vi "edit_configurations.vi"() -> ()   [LabVIEW 2010]
uses:
  main/labview_source/type_definitions/classes/GenericPlugin/GenericPlugin.lvclass
  main/labview_source/type_definitions/clusters/plugin_specification.ctl
panel:
  in  "new":bool
  in  "Name":string
  in  "configure":bool
  in  "done":bool
  in  "Configuration":string(combo)
  in  "Path":path
  # "Edit existing configuration"
  # "create new configuration"
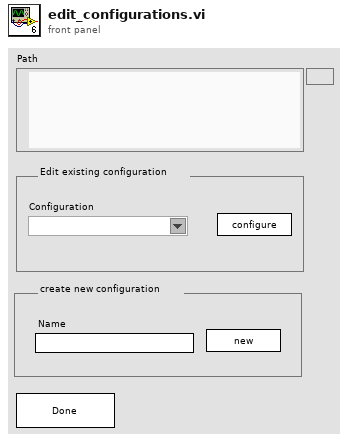
[diagram p1: front panel]
types:
  T1 = typedef "plugin_specification.ctl" = cluster{"class path":path, "configuration":string, "label":string}
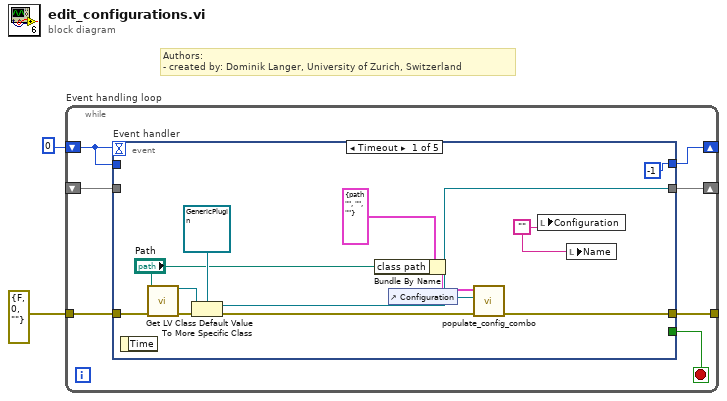
[diagram p0: block diagram]
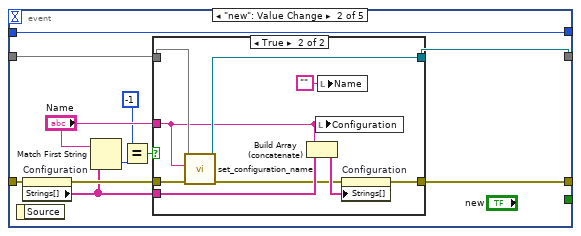
[diagram p2: hidden frame]
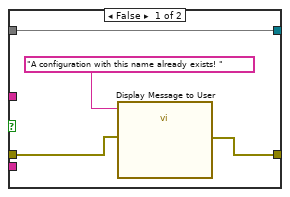
[diagram p3: hidden frame]
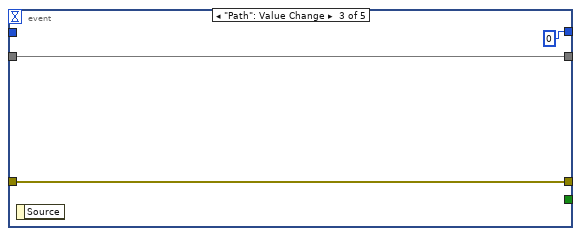
[diagram p4: hidden frame]
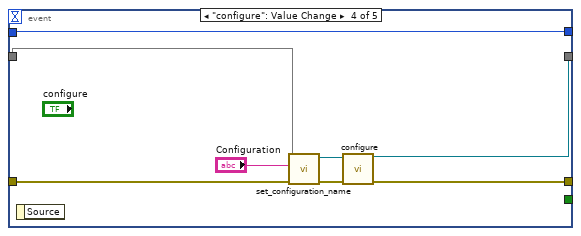
[diagram p5: hidden frame]
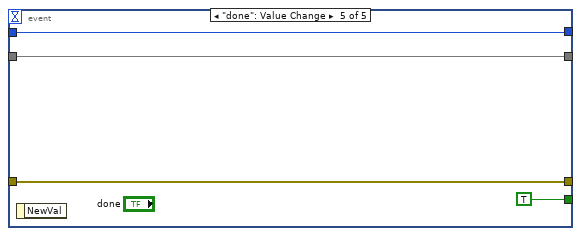
[diagram p6: hidden frame]
diagram:
  # "Authors: \n- created by: Dominik Langer, University of Zurich, Switzerland"
  n1 = while "Event handling loop" {
    shift-right: [w8] -> _
    shift-left: 0 -> [w9]
    shift-right: [w5] -> _
    shift-left: _ -> [w4]
    tunnel: errorcluster {"status"=FALSE, "code"=0, "source"=""} ("error in (no error)") -> [w6]
    tunnel: [w3] -> _
    stop <- w7 stop-if-true
    n2 = event "Event handler" shown="[0] Timeout" {
      selector: _ -> [_ _ _ _ _]
      dyn-events: _ -> [_ _ _ _ _]
      timeout: w9 -> [_ _ _ _ _]
      tunnel: w9 -> [_ w30 _ w52 w61]
      tunnel: [-1 w30 0 w52 w61] -> w8
      tunnel: [_ _ _ _ TRUE] -> w7
      tunnel: w6 -> [w21 w29 w47 w57 w58]
      tunnel: [w17 w32 w48 w53 w59] -> w5
      tunnel: w4 -> [_ w33 w48 w55 w59]
      tunnel: [w15 w31 w47 w51 w58] -> w3
      event Timeout {
        w16 = ""
        n3 = event-data() -> ()  [unwired: 2 out]
        n4 = call <vilib>:"Get LV Class Default Value.vi"("error in (no error)"=w21, "class path"="Path") -> ("error out"=w20:errorcluster, "object"=w19:refnum<class>)  [unwired: 8 out]
        n5 = To More Specific Class(target class=refnum<class "GenericPlugin.lvclass"> refnum ("GenericPlugin.lvclass"), reference=w19, error in=w20) -> (specific class reference=w17:refnum<class "GenericPlugin.lvclass">, error out=w14:errorcluster)
        n6 = Bundle By Name(cluster=T1 {"class path"=path "", "configuration"="", "label"=""} ("plug-in specification"), "class path"="Path") -> (w11:T1)
        n7 = control-ref of="Configuration"() -> (w13:refnum<vi>)
        n8 = call "populate_config_combo.vi"("error in (no error)"=w14, "combo-box reference"=w13, "plug-in specification"=w11) -> ("error out"=w15:errorcluster)  [unwired: 8 out]
        n9 = local write "Configuration"(w16) -> ()
        n10 = local write "Name"(w16) -> ()
      }
      event "new": Value Change {
        n11 = event-data() -> ()  [unwired: 2 out]
        n12 = property on="Configuration" class="CmbBox"(error in=w29) -> (error out=w28:errorcluster, "Strings[]"=w27:string[])  [unwired: 1 in, 1 out]
        n13 = Match First String(2:w27, 3:"Name") -> (0:w25:i32)  [unwired: 1 out]
        n14 = Equal?(x=-1, y=w25) -> (x = y?=w24:bool)
        n15 = case shown="True" w24 {
          tunnel: w28 -> [w36 w46]
          tunnel: w33 -> [w37 w45]
          tunnel: [w37 w44] -> w32
          tunnel: [w35 w43] -> w31
          tunnel: "Name" -> [_ w41]
          tunnel: w27 -> [_ w40]
          frame False {
            n16 = call "Display Message to User"("error in (no error)"=w36, "Message"="A configuration with this name already exists! ") -> ("error out"=w35:errorcluster)  [unwired: 1 in, 8 out]
          }
          frame True {
            n17 = call-dynamic "set_configuration_name.vi"("error in (no error)"=w46, "configuration"=w41, "GenericPlugin.lvclass in"=w45) -> ("error out"=w38:errorcluster, "GenericPlugin.lvclass out"=w44:refnum<class "GenericPlugin.lvclass">)  [unwired: 7 out]
            n18 = Build Array (concatenate)(w41, w40) -> (w42:string[])
            n19 = local write "Configuration"(w41) -> ()
            n20 = local write "Name"("") -> ()
            n21 = property on="Configuration" class="CmbBox"(error in=w38, "Strings[]"=w42) -> (error out=w43:errorcluster)  [unwired: 1 in, 1 out]
          }
        }
      }
      event "Path": Value Change {
        n22 = event-data() -> ()  [unwired: 2 out]
      }
      event "configure": Value Change {
        n23 = event-data() -> ()  [unwired: 2 out]
        n24 = call-dynamic "set_configuration_name.vi"("error in (no error)"=w57, "configuration"="Configuration", "GenericPlugin.lvclass in"=w55) -> ("error out"=w56:errorcluster, "GenericPlugin.lvclass out"=w54:refnum<class "GenericPlugin.lvclass">)  [unwired: 7 out]
        n25 = call-dynamic "configure.vi"("error in (no error)"=w56, "GenericPlugin in"=w54) -> ("error out"=w51:errorcluster, "GenericPlugin out"=w53:refnum<class "GenericPlugin.lvclass">)  [unwired: 8 out]
      }
      event "done": Value Change {
        n26 = event-data() -> ()  [unwired: 2 out]
      }
    }
  }
